vi "ContBuildProgamQueue.vi"(10 "Continuous Program":string[][](array[string]), 11 "queue in":refnum<queue>) -> (3 "queue out":refnum<queue>)   [LabVIEW 2018]
uses:
  <vilib>/regexp/Match Regular Expression.xnode
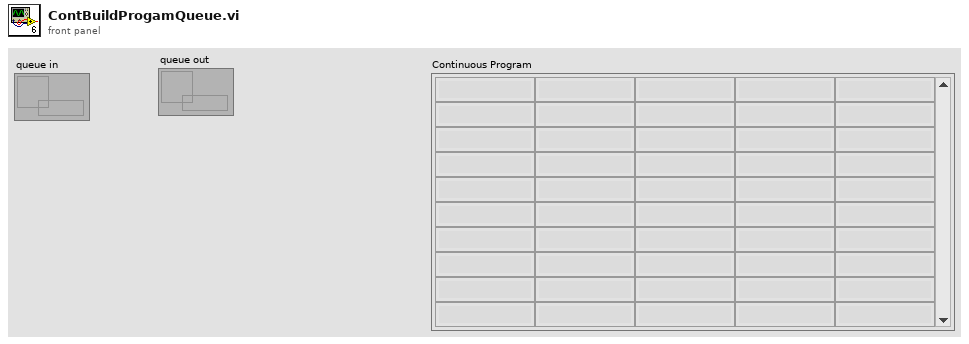
[diagram p1: front panel]
types:
  T1 = cluster{"Step Name":string, "Time":variant, "Param 1":variant, "Param 2":variant}
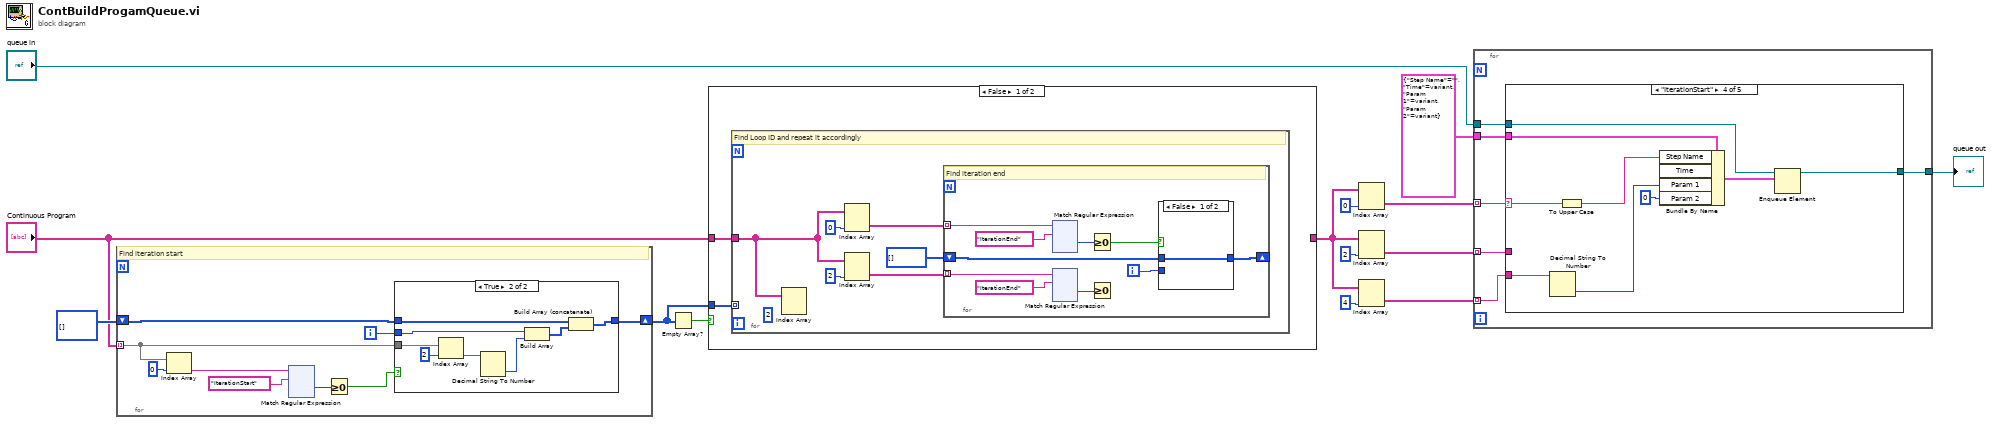
[diagram p0: block diagram]
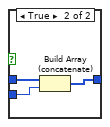
[diagram p2: hidden frame]
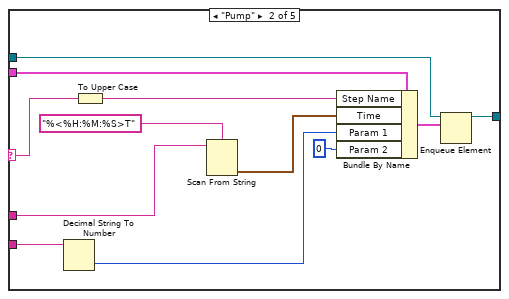
[diagram p6: hidden frame]
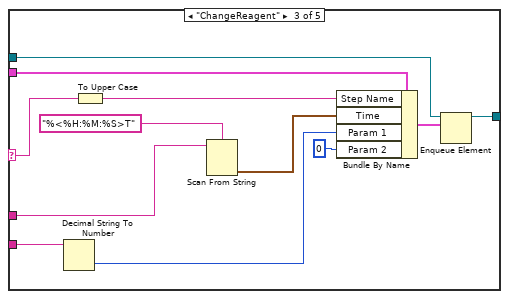
[diagram p7: hidden frame]
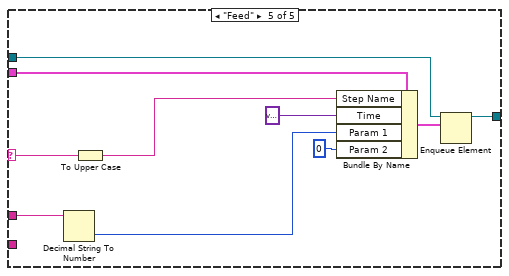
[diagram p8: hidden frame]
diagram:
  n1 = for {
    shift-right: [w20] -> w2
    shift-left: i32[][] [] -> [w19]
    tunnel: "Continuous Program" -> [w16] mode=indexing
    i -> [w15]
    # "Find iteration start"
    n2 = Index Array(array=w16, index=0 ("disabled index (col)")) -> (element=w18:string)
    n3 = xnode "Match Regular Expression"("input string"=w18, "regular expression"="IterationStart" ("element")) -> ("offset past match"=w22:i32)  [unwired: 4 in, 4 out]
    n4 = Greater Or Equal To 0?(x=w22) -> (x >= 0?=w21:bool)
    n5 = case shown="True" w21 {
      tunnel: [w24 w32] -> w20
      tunnel: w19 -> [w24 w31]
      tunnel: w16 -> [_ w29]
      tunnel: w15 -> [_ w26]
      frame False {
      }
      frame True {
        n6 = Index Array(array=w29, index=2 ("disabled index (col)")) -> (element=w28:string)
        n7 = Decimal String To Number(string=w28) -> (number=w27:i32)  [unwired: 2 in, 1 out]
        n8 = Build Array(w26, w27) -> (w25:i32[])
        n9 = Build Array (concatenate)(w31, w25) -> (w32:i32[][])
      }
    }
  }
  n10 = Empty Array?(array=w2) -> (empty?=w4:bool)
  n11 = case shown="False" w4 {
    tunnel: "Continuous Program" -> [w147 w397]
    tunnel: [_ w397] -> w3
    tunnel: w2 -> [w148 _]
    frame False {
      n12 = for {
        tunnel: w148 -> [_] mode=indexing
        tunnel: w147 -> [w150]
        (unwired) 2 ("disabled index (col)")
        # "Find Loop ID and repeat it accordingly"
        n13 = Index Array(array=w150) -> ()  [unwired: 2 in, 1 out]
        n14 = Index Array(array=w150, index (col)=0 ("disabled index (col)")) -> (element=w152:string[])  [unwired: 1 in]
        n15 = Index Array(array=w150, index (col)=2 ("disabled index (col)")) -> (element=w149:string[])  [unwired: 1 in]
        n16 = for {
          tunnel: w152 -> [w164] mode=indexing
          shift-right: [w160] -> _
          shift-left: i32[] [] -> [w159]
          tunnel: w149 -> [w155] mode=indexing
          i -> [w158]
          # "Find iteration end"
          n17 = xnode "Match Regular Expression"("input string"=w164, "regular expression"="IterationEnd" ("element")) -> ("offset past match"=w162:i32)  [unwired: 4 in, 4 out]
          n18 = xnode "Match Regular Expression"("input string"=w155, "regular expression"="IterationEnd" ("element")) -> ("offset past match"=w156:i32)  [unwired: 4 in, 4 out]
          n19 = Greater Or Equal To 0?(x=w162) -> (x >= 0?=w161:bool)
          n20 = Greater Or Equal To 0?(x=w156) -> ()  [unwired: 1 out]
          n21 = case shown="False" w161 {
            tunnel: [w279 w282] -> w160
            tunnel: w159 -> [w279 w281]
            tunnel: w158 -> [_ w280]
            frame False {
            }
            frame True {
              n22 = Build Array (concatenate)(w281, w280) -> (w282:i32[])
            }
          }
        }
      }
    }
    frame True {
    }
  }
  n23 = Index Array(array=w3, index (col)=0 ("disabled index (col)")) -> (element=w14:string[])  [unwired: 1 in]
  n24 = Index Array(array=w3, index (col)=2 ("disabled index (col)")) -> (element=w11:string[])  [unwired: 1 in]
  n25 = Index Array(array=w3, index (col)=4 ("disabled index (col)")) -> (element=w9:string[])  [unwired: 1 in]
  n26 = for {
    tunnel: w14 -> [w401] mode=indexing
    tunnel: w11 -> [w403] mode=indexing
    tunnel: w9 -> [w402] mode=indexing
    tunnel: T1 {"Step Name"="", "Time"=variant, "Param 1"=variant, "Param 2"=variant} -> [w400]
    tunnel: [w399] -> w7
    tunnel: "queue in" -> [w398]
    n27 = case shown="\"IterationStart\"" w401 {
      selector: w401 -> [_ w409 w421 w433 w437]
      tunnel: w403 -> [_ w414 w426 _ w446]
      tunnel: w402 -> [_ w415 w427 w436 _]
      tunnel: w400 -> [_ w412 w424 w435 w441]
      tunnel: [_ w406 w418 w430 w440] -> w399
      tunnel: w398 -> [_ w405 w417 w429 w439]
      frame Default {
      }
      frame "Pump" {
        n28 = Decimal String To Number(string=w415) -> (number=w411:i32)  [unwired: 2 in, 1 out]
        n29 = To Upper Case(1:w409) -> (0:w404:string)
        n30 = Scan From String(format string="%<%H:%M:%S>T", input string=w414) -> (output 1=w410:timestamp)  [unwired: 3 in, 3 out]
        n31 = Bundle By Name(cluster=w412, "Step Name"=w404, "Time"=w410, "Param 1"=w411, "Param 2"=0) -> (w408:T1)
        n32 = Enqueue Element(queue=w405, element=w408) -> (queue out=w406:refnum<queue>)  [unwired: 2 in, 2 out]
      }
      frame "ChangeReagent" {
        n33 = Decimal String To Number(string=w427) -> (number=w423:i32)  [unwired: 2 in, 1 out]
        n34 = To Upper Case(1:w421) -> (0:w416:string)
        n35 = Scan From String(format string="%<%H:%M:%S>T", input string=w426) -> (output 1=w422:timestamp)  [unwired: 3 in, 3 out]
        n36 = Bundle By Name(cluster=w424, "Step Name"=w416, "Time"=w422, "Param 1"=w423, "Param 2"=0) -> (w420:T1)
        n37 = Enqueue Element(queue=w417, element=w420) -> (queue out=w418:refnum<queue>)  [unwired: 2 in, 2 out]
      }
      frame "IterationStart" {
        n38 = Decimal String To Number(string=w436) -> (number=w434:i32)  [unwired: 2 in, 1 out]
        n39 = To Upper Case(1:w433) -> (0:w428:string)
        n40 = Bundle By Name(cluster=w435, "Step Name"=w428, "Param 1"=w434, "Param 2"=0) -> (w432:T1)  [unwired: 1 in]
        n41 = Enqueue Element(queue=w429, element=w432) -> (queue out=w430:refnum<queue>)  [unwired: 2 in, 2 out]
      }
      frame "Feed" {
        n42 = Decimal String To Number(string=w446) -> (number=w443:i32)  [unwired: 2 in, 1 out]
        n43 = To Upper Case(1:w437) -> (0:w438:string)
        n44 = Bundle By Name(cluster=w441, "Step Name"=w438, "Time"=variant, "Param 1"=w443, "Param 2"=0) -> (w445:T1)
        n45 = Enqueue Element(queue=w439, element=w445) -> (queue out=w440:refnum<queue>)  [unwired: 2 in, 2 out]
      }
    }
  }
  "queue out" <- w7
